vi "run top level.vi"(8 "results reporter":refnum<class "results reporter.lvclass">, 9 "execution system":T1=enum."standard", 10 "thread pool":refnum<class "thread pool.lvclass">, 11 "task":refnum<class "task.lvclass">) -> ()   [LabVIEW 2014, in "task.lvclass"]
uses:
  task.lvclass
  dispatcher/thread pool.lvclass
  dispatcher/execution system.ctl
  results reporter/results reporter.lvclass
  result/result.lvclass
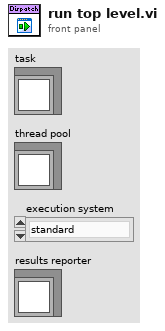
[diagram p1: front panel]
types:
  T1 = typedef "thread pool.lvclass/execution system.ctl" = enum32{"user interface", "standard", "instrument i/o", "data acquisition", "other 1", "other 2"}
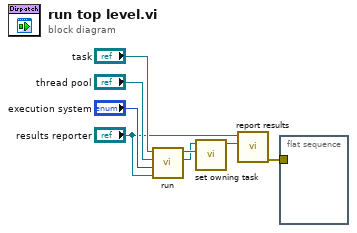
[diagram p0: block diagram]
diagram:
  n1 = call-dynamic "run.vi"("results reporter"="results reporter", "execution system"="execution system", "thread pool"="thread pool", "task in"="task") -> ("result"=w5:refnum<class "result.lvclass">, "task out"=w6:refnum<class "task.lvclass">)  [unwired: 6 in]
  n2 = call "set owning task.vi"("task"=w6, "result in"=w5) -> ("result out"=w4:refnum<class "result.lvclass">)  [unwired: 9 in]
  n3 = call-dynamic "report results.vi"("result"=w4, "results reporter in"="results reporter") -> ("error out"=w7:errorcluster)  [unwired: 8 in, 1 out]
  n4 = flat-sequence {
    tunnel: w7 -> [_]
    frame #0 {
    }
  }
